vi "read.vi"(9 "continuation timeout (10000)":i32=-1, 10 "base timeout (5000)":i32=-1, 11 "websocket client in":refnum<class "websocket client.lvclass">) -> (0 "error out":errorcluster, 1 "Numeric":u8=2, 2 "message":string, 3 "websocket client out":refnum<class "websocket client.lvclass">)   [LabVIEW 2016, in "websocket client.lvclass"]
uses:
  websocket client.lvclass
  websocket client.lvclass/websocket client.ctl
  websocket core.lvlib
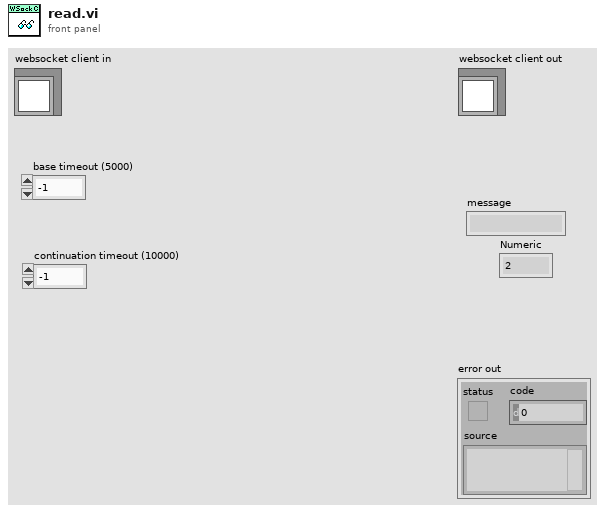
[diagram p1: front panel]
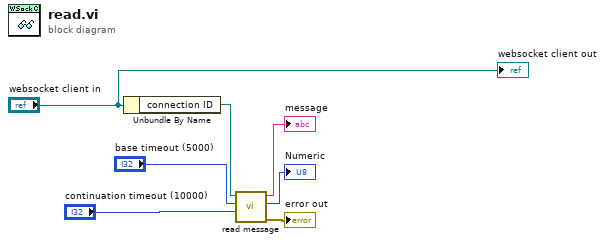
[diagram p0: block diagram]
diagram:
  n1 = Unbundle By Name("websocket client in") -> ("connection ID"=w6:refnum<k5>)
  n2 = call "read message.vi"("continuation timeout (10000)"="continuation timeout (10000)", "base timeout (5000)"="base timeout (5000)", "tcp connection"=w6) -> ("error"=→"error out":errorcluster, "Numeric"=→"Numeric":u8, "message"=→"message":string)  [unwired: 6 in]
  "websocket client out" <- "websocket client in"
